vi "close_matflie.vi"(8 "error in":errorcluster, 11 "matFile_info IN":T1) -> (0 "error out":errorcluster, 3 "matFile_info OUT":T1)   [LabVIEW 2018]
uses:
  MatFile_information.ctl
  type_control.ctl
panel:
  out "col":i32[](array[numeric])
  out "row":i32[](array[numeric])
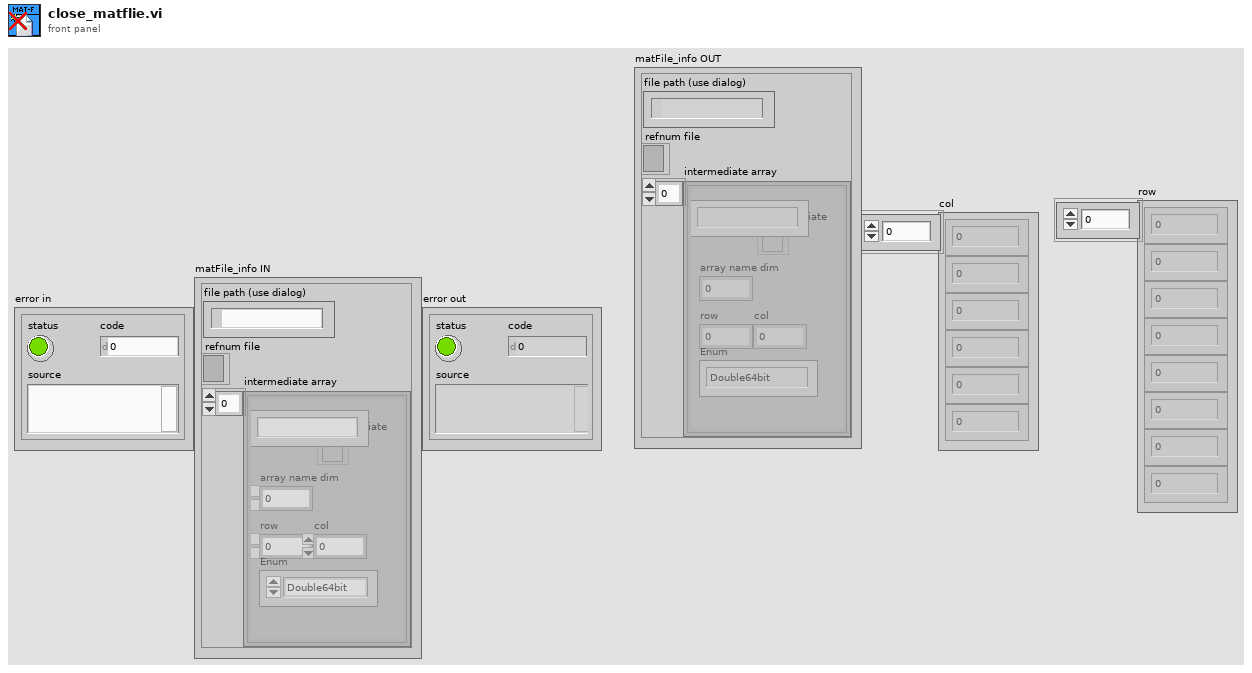
[diagram p1: front panel]
types:
  T1 = typedef "MatFile_information.ctl" = cluster{"file path (use dialog)":path, "refnum file":refnum<file>, "intermediate array":cluster{"intermediate":refnum<file>, "array name dim":i32, "row":i32, "col":i32, "Content":string, "Enum":T2}[]}
  T2 = typedef "type_control.ctl" = enum16{"Int8bit_elem", "Int8bit", "Int64bit_elem", "Int64bit", "Int16bit_elem", "Double64bit_elem", "Int16bit", "Double64bit"}
  T3 = enum16{"big-endian, network order", "native, host order", "little-endian"}
  T4 = cluster{"intermediate":refnum<file>, "array name dim":i32, "row":i32, "col":i32, "Content":string, "Enum":T2}[]
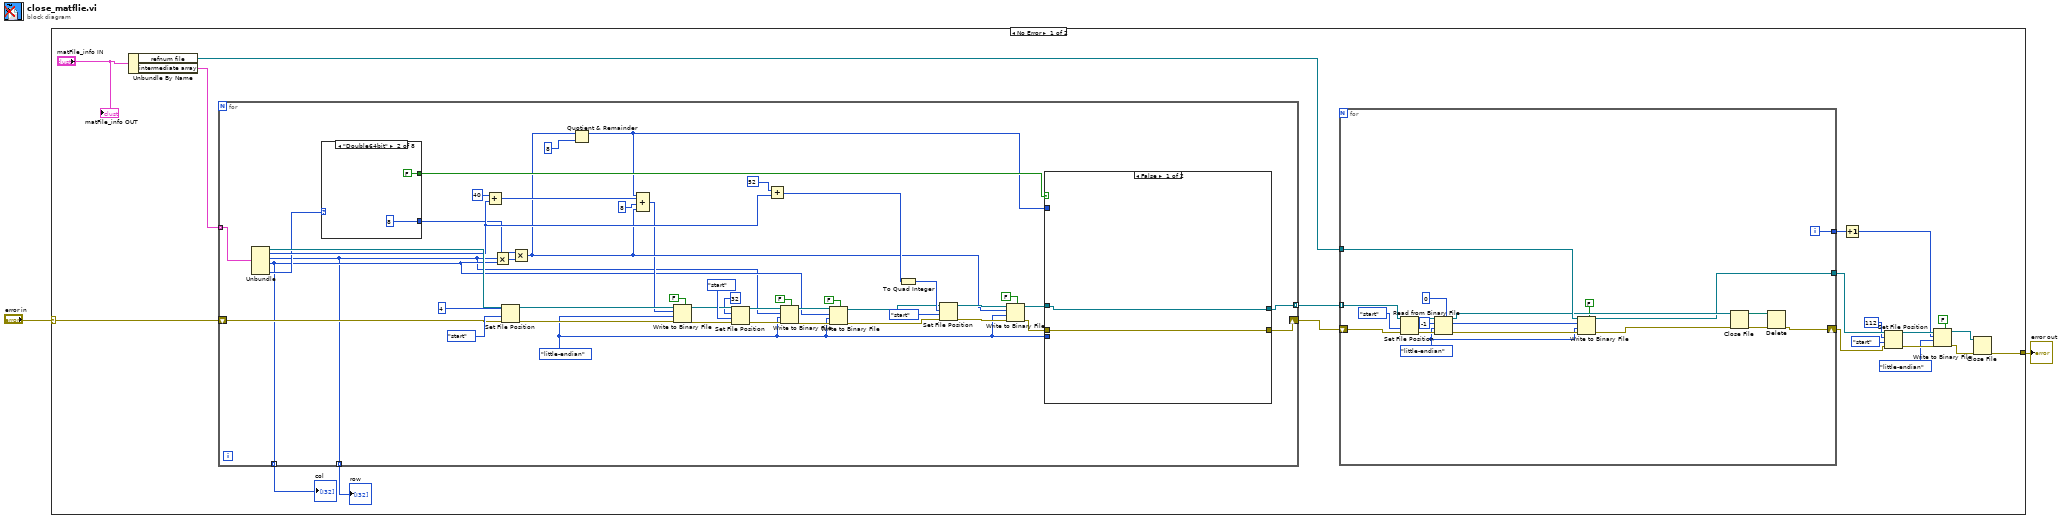
[diagram p0: block diagram]
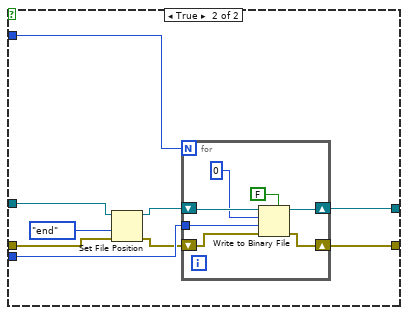
[diagram p2: hidden frame]
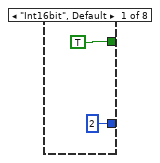
[diagram p3: hidden frame]
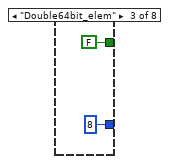
[diagram p4: hidden frame]
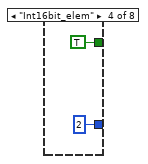
[diagram p5: hidden frame]
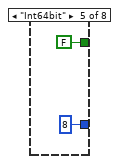
[diagram p6: hidden frame]
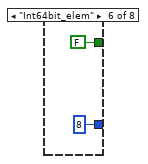
[diagram p7: hidden frame]
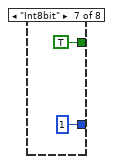
[diagram p8: hidden frame]
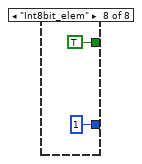
[diagram p9: hidden frame]
diagram:
  n1 = case shown="No Error" "error in" {
    selector: "error in" -> [w21 w123]
    tunnel: [w18 w123] -> w1
    frame No Error {
      n2 = Unbundle By Name("matFile_info IN") -> ("refnum file"=w19:refnum<file>, "intermediate array"=w22:T4)
      n3 = for {
        tunnel: w22 -> [w88] mode=indexing
        shift-right: [w55] -> w20
        shift-left: w21 -> [w86]
        tunnel: [w53] -> w17 mode=indexing
        tunnel: [w44] -> w16 mode=indexing
        tunnel: [w43] -> w15 mode=indexing
        w54 = T3."little-endian" ("byte order (0:big-endian, network order)")
        n4 = Unbundle(w88) -> ("intermediate"=w84:refnum<file>, "array name dim"=w65:i32, "row"=w43:i32, "col"=w44:i32, "Enum"=w58:T2)  [unwired: 1 out]
        n5 = case shown="\"Double64bit\"" w58 {
          tunnel: [2 8 8 2 8 8 1 1] -> w52
          tunnel: [TRUE FALSE FALSE TRUE FALSE FALSE TRUE TRUE] -> w50
          frame "Int16bit", Default {
          }
          frame "Double64bit" {
          }
          frame "Double64bit_elem" {
          }
          frame "Int16bit_elem" {
          }
          frame "Int64bit" {
          }
          frame "Int64bit_elem" {
          }
          frame "Int8bit" {
          }
          frame "Int8bit_elem" {
          }
        }
        n6 = Add(x=40, y=w65) -> (x+y=w48:i32)
        n7 = Multiply(x=w43, y=w44) -> (x*y=w81:i32)
        n8 = Set File Position(offset (in bytes) (0)=i64 4, refnum=w84, from (0:start)=enum16{"start", "end", "current"}."start", error in=w86) -> (refnum out=w80:refnum<file>, error out=w83:errorcluster)
        n9 = Multiply(x=w52, y=w81) -> (x*y=w46:i32)
        n10 = Quotient & Remainder(x=w46, y=8) -> (x-y*floor(x/y)=w49:i32)  [unwired: 1 out]
        n11 = Compound Arithmetic op=ADD(w49, w48, 8 ("value"), w46) -> (w45:i32)
        n12 = Write to Binary File(file (use dialog)=w80, data=w45, error in=w83, 5:FALSE ("prepend array or string size? (T)"), 9:w54) -> (refnum out=w72:refnum<file>, error out=w71:errorcluster)  [unwired: 1 in, 1 out]
        n13 = Set File Position(offset (in bytes) (0)=i64 32, refnum=w72, from (0:start)=enum16{"start", "end", "current"}."start", error in=w71) -> (refnum out=w67:refnum<file>, error out=w68:errorcluster)
        n14 = Add(x=52, y=w65) -> (x+y=w64:i32)
        n15 = Write to Binary File(file (use dialog)=w67, data=w43, error in=w68, 5:FALSE ("prepend array or string size? (T)"), 9:w54) -> (refnum out=w60:refnum<file>, error out=w61:errorcluster)  [unwired: 1 in, 1 out]
        n16 = Write to Binary File(file (use dialog)=w60, data=w44, error in=w61, 5:FALSE ("prepend array or string size? (T)"), 9:w54) -> (refnum out=w59:refnum<file>, error out=w62:errorcluster)  [unwired: 1 in, 1 out]
        n17 = To Quad Integer(1:w64) -> (0:w77:i64)
        n18 = Set File Position(offset (in bytes) (0)=w77, refnum=w59, from (0:start)=enum16{"start", "end", "current"}."start", error in=w62) -> (refnum out=w74:refnum<file>, error out=w75:errorcluster)
        n19 = Write to Binary File(file (use dialog)=w74, data=w46, error in=w75, 5:FALSE ("prepend array or string size? (T)"), 9:w54) -> (refnum out=w56:refnum<file>, error out=w57:errorcluster)  [unwired: 1 in, 1 out]
        n20 = case shown="False" w50 {
          tunnel: w57 -> [w89 w95]
          tunnel: w56 -> [w90 w92]
          tunnel: w49 -> [_ w91]
          tunnel: [w89 w99] -> w55
          tunnel: w54 -> [_ w98]
          tunnel: [w90 w97] -> w53
          frame False {
          }
          frame True {
            n21 = Set File Position(refnum=w92, from (0:start)=enum16{"start", "end", "current"}."end", error in=w95) -> (refnum out=w93:refnum<file>, error out=w94:errorcluster)  [unwired: 1 in]
            n22 = for {
              N: w91 -> [_]
              shift-right: [w105] -> w99
              shift-left: w94 -> [w104]
              tunnel: w98 -> [w103]
              shift-right: [w100] -> w97
              shift-left: w93 -> [w102]
              n23 = Write to Binary File(file (use dialog)=w102, data=i8 0, error in=w104, 5:FALSE ("prepend array or string size? (T)"), 9:w103) -> (refnum out=w100:refnum<file>, error out=w105:errorcluster)  [unwired: 1 in, 1 out]
            }
          }
        }
      }
      "col" <- w16
      "row" <- w15
      n24 = for {
        shift-right: [w27] -> w7
        shift-left: w20 -> [w41]
        tunnel: w19 -> [w36]
        tunnel: [w33] -> w10
        tunnel: w17 -> [w26] mode=indexing
        tunnel: [w24] -> w5
        i -> [w24]
        w25 = T3."little-endian" ("byte order (0:big-endian, network order)")
        n25 = Set File Position(refnum=w26, from (0:start)=enum16{"start", "end", "current"}."start", error in=w41) -> (refnum out=w39:refnum<file>, error out=w40:errorcluster)  [unwired: 1 in]
        n26 = Read from Binary File(5:i64 0 ("Numeric"), 8:w40, 9:w25, 10:-1 ("count (1)"), 11:w39) -> (0:w38:errorcluster, 2:w37:i64[], 3:w34:refnum<file>)  [unwired: 1 in, 1 out]
        n27 = Write to Binary File(file (use dialog)=w36, data=w37, error in=w38, 5:FALSE ("prepend array or string size? (T)"), 9:w25) -> (refnum out=w33:refnum<file>, error out=w35:errorcluster)  [unwired: 1 in, 1 out]
        n28 = Close File(refnum=w34, error in=w35) -> (path=w28:path, error out=w29:errorcluster)
        n29 = Delete(path (use dialog)=w28, error in=w29) -> (error out=w27:errorcluster)  [unwired: 3 in, 2 out]
      }
      n30 = Increment(x=w5) -> (x+1=w4:i32)
      n31 = Set File Position(offset (in bytes) (0)=i64 112, refnum=w10, from (0:start)=enum16{"start", "end", "current"}."start", error in=w7) -> (refnum out=w11:refnum<file>, error out=w12:errorcluster)
      n32 = Write to Binary File(file (use dialog)=w11, data=w4, error in=w12, 5:FALSE ("prepend array or string size? (T)"), 9:T3."little-endian" ("byte order (0:big-endian, network order)")) -> (refnum out=w13:refnum<file>, error out=w14:errorcluster)  [unwired: 1 in, 1 out]
      n33 = Close File(refnum=w13, error in=w14) -> (error out=w18:errorcluster)  [unwired: 1 out]
      "matFile_info OUT" <- "matFile_info IN"
    }
    frame Error {
    }
  }
  "error out" <- w1
